vi "Create Data Channels.vi"(8 "error in":errorcluster, 11 "Node in":refnum<class "AMS Chiller Template.lvclass">) -> (0 "error out":errorcluster, 3 "Node out":refnum<class "AMS Chiller Template.lvclass">)   [LabVIEW 2026, in "AMS Chiller Template.lvlib" / "AMS Chiller Template.lvclass"]
uses:
  AMS Chiller Template.lvclass
  <vilib>/ADAS Replay HIL/Template Node/Plugin/Template Node/Template Node.lvclass/Template Node.ctl
  AMS Chiller Template.lvclass/AMS Chiller Template.ctl
  C:/Program Files/National Instruments/AMS plugin/Capabilities/Capabilities/High Level Capabilities/Chiller Cluster/Chiller Cluster.lvclass
  <vilib>/ADAS Replay HIL/Template Node/Plugin/Template Node/Template Node.lvclass
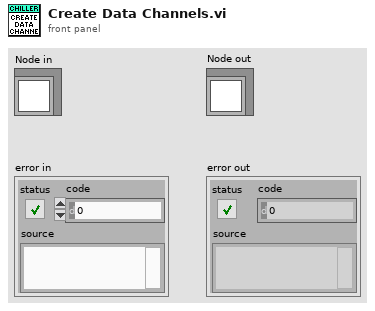
[diagram p1: front panel]
types:
  T1 = typedef "AMS Chiller Template.lvlib/AMS Chiller Template.lvclass/Configuration Params.ctl" = cluster{"Common":T2, "Amount of Channels":u32, "Address":string}
  T2 = typedef "Template Node.lvlib/Template Node.lvclass/Common Configuration Params.ctl" = cluster{"Iteration Interval (s)":dbl, "T0 (ns)":u64, "Priority":i32, "Processor":i32, "Wait in Ready State":bool}
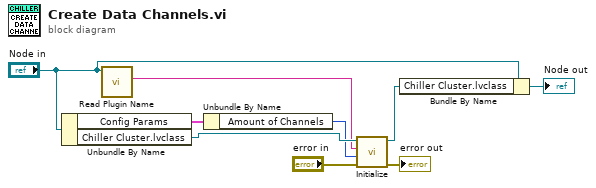
[diagram p0: block diagram]
diagram:
  n1 = Unbundle By Name("Node in") -> ("Config Params"=w9:T1, "Chiller Cluster.lvclass"=w5:refnum<class "Chiller Cluster.lvclass">)
  n2 = call <vilib>:"Read Plugin Name.vi"("Template Node in"="Node in") -> ("Plugin Name"=w4:string)  [unwired: 8 in, 2 out]
  n3 = Unbundle By Name(w9) -> ("Amount of Channels"=w3:u32)
  n4 = call-dynamic "Initialize.vi"("error in"="error in", "Channels Amount"=w3, "InstanceName"=w4, "Chiller Cluster.lvclass in"=w5) -> ("error out"=→"error out":errorcluster, "Chiller Cluster.lvclass out"=w6:refnum<class "Chiller Cluster.lvclass">)  [unwired: 6 in]
  n5 = Bundle By Name(cluster="Node in", "Chiller Cluster.lvclass"=w6) -> (→"Node out":refnum<class "AMS Chiller Template.lvclass">)
